vi "FTW_AppLauncher-Core_Config_Populate.vi"(0 "FTW-AppLauncher-Core In":refnum<class "FTW-AppLauncher-Core.lvclass">, 11 "error in":errorcluster) -> (4 "FTW-AppLauncher-Core Out":refnum<class "FTW-AppLauncher-Core.lvclass">, 6 "Configuration String":string, 15 "error out":errorcluster)   [LabVIEW 2013, in "FTW-AppLauncher-Core.lvclass"]
uses:
  FTW-AppLauncher-Core.lvclass
  source/JSON/FTW-JSON-UpdateMode.ctl
  FTW-AppLauncher-Core.lvclass/FTW-AppLauncher-Core.ctl
  source/JSON/FTW-JSON.lvclass
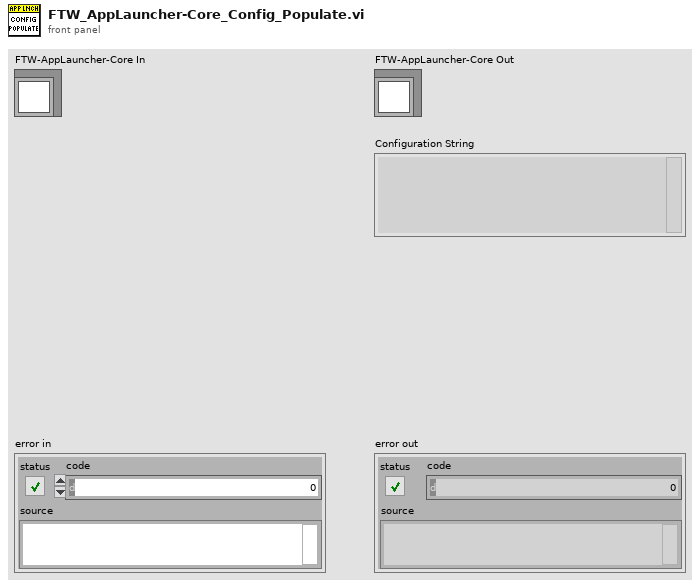
[diagram p1: front panel]
types:
  T1 = typedef "FTW-JSON.lvclass/FTW-JSON-UpdateMode.ctl" = enum16{"Upsert", "Update Only", "Insert Only"}
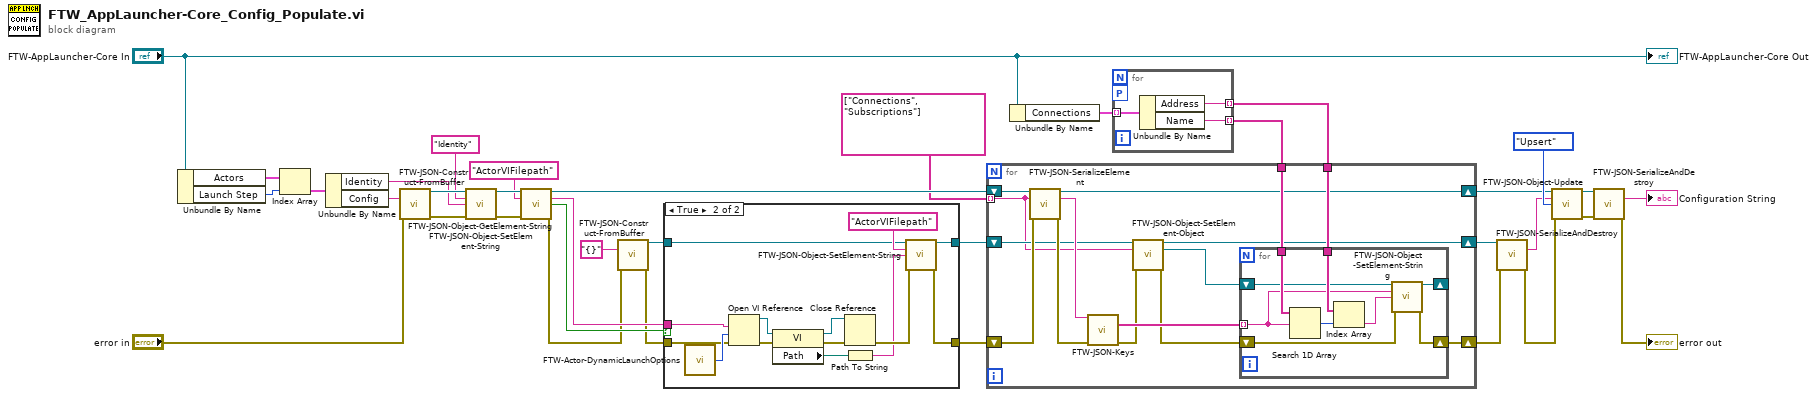
[diagram p0: block diagram]
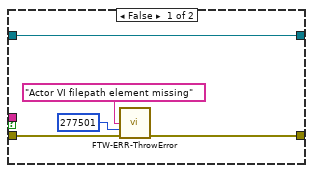
[diagram p2: hidden frame]
diagram:
  n1 = Unbundle By Name("FTW-AppLauncher-Core In") -> ("Actors"=w36:cluster{"Identity":string, "Config":string}[], "Launch Step"=w35:i32)
  n2 = Index Array(array=w36, index=w35) -> (element=w34:cluster{"Identity":string, "Config":string})
  n3 = Unbundle By Name(w34) -> ("Identity"=w30:string, "Config"=w22:string)
  n4 = call "FTW-JSON-Construct-FromBuffer.vi"("JSON String (UTF-8)"=w22, "error in"="error in") -> ("JSON Object"=w33:refnum<class "FTW-JSON.lvclass">, "error out"=w32:errorcluster)  [unwired: 12 in]
  n5 = call "FTW-JSON-Object-SetElement-String.vi"("JSON Object"=w33, "Key"="Identity", "Value"=w30, "error in"=w32) -> ("JSON Object out"=w29:refnum<class "FTW-JSON.lvclass">, "error out"=w28:errorcluster)  [unwired: 10 in]
  n6 = call "FTW-JSON-Object-GetElement-String.vi"("JSON Object"=w29, "Key"="ActorVIFilepath", "error in"=w28) -> ("JSON Object out"=w20:refnum<class "FTW-JSON.lvclass">, "Value"=w26:string, "Found?"=w21:bool, "error out"=w6:errorcluster)  [unwired: 9 in]
  n7 = call "FTW-JSON-Construct-FromBuffer.vi"("JSON String (UTF-8)"="{}", "error in"=w6) -> ("JSON Object"=w7:refnum<class "FTW-JSON.lvclass">, "error out"=w5:errorcluster)  [unwired: 12 in]
  n8 = case shown="True" w21 {
    tunnel: w26 -> [_ w49]
    tunnel: [w37 w43] -> w17
    tunnel: [w38 w44] -> w23
    tunnel: w5 -> [w39 w45]
    tunnel: w7 -> [w37 w42]
    frame False {
      n9 = call "FTW-ERR-ThrowError.vi"("Error Message"="Actor VI filepath element missing", "Error Code"=277501, "error in"=w39) -> ("error out"=w38:errorcluster)  [unwired: 12 in]
    }
    frame True {
      n10 = call "FTW-Actor-DynamicLaunchOptions.vi"() -> ("Open VI Ref Options"=w55:i32)
      n11 = Open VI Reference(vi path=w49, options=w55, error in (no error)=w45) -> (vi reference=w52:refnum<vi>, error out=w54:errorcluster)  [unwired: 3 in]
      n12 = property class="VI"(reference=w52, error in=w54) -> (reference out=w51:refnum<vi>, error out=w53:errorcluster, "Path"=w50:path)
      n13 = Close Reference(reference=w51, error in (no error)=w53) -> (error out=w48:errorcluster)
      n14 = Path To String(path=w50) -> (string=w46:string)
      n15 = call "FTW-JSON-Object-SetElement-String.vi"("JSON Object"=w42, "Key"="ActorVIFilepath", "Value"=w46, "error in"=w48) -> ("JSON Object out"=w43:refnum<class "FTW-JSON.lvclass">, "error out"=w44:errorcluster)  [unwired: 10 in]
    }
  }
  n16 = Unbundle By Name("FTW-AppLauncher-Core In") -> ("Connections"=w18:cluster{"Name":string, "Address":string}[])
  n17 = for {
    tunnel: w18 -> [w58] mode=indexing
    workers-P: _ -> [_]
    tunnel: [w57] -> w15 mode=indexing
    tunnel: [w56] -> w16 mode=indexing
    n18 = Unbundle By Name(w58) -> ("Address"=w56:string, "Name"=w57:string)
  }
  n19 = for {
    tunnel: string[] ["Connections", "Subscriptions"] -> [w61] mode=indexing
    tunnel: w16 -> [w67]
    tunnel: w15 -> [w66]
    shift-right: [w59] -> w4
    shift-left: w17 -> [w62]
    shift-right: [w64] -> w3
    shift-left: w23 -> [w73]
    shift-right: [w65] -> w14
    shift-left: w20 -> [w71]
    n20 = call "FTW-JSON-SerializeElement.vi"("JSON Object"=w71, "Key"=w61, "error in"=w73) -> ("JSON Object"=w65:refnum<class "FTW-JSON.lvclass">, "Element as JSON String"=w70:string, "error out"=w72:errorcluster)  [unwired: 9 in, 1 out]
    n21 = call "FTW-JSON-Keys.vi"("JSON Opject"=w70, "error in"=w72) -> ("Keys"=w69:string[], "error out"=w68:errorcluster)  [unwired: 11 in, 1 out]
    n22 = call "FTW-JSON-Object-SetElement-Object.vi"("JSON Object"=w62, "Key"=w61, "error in"=w68) -> ("JSON Root Object"=w59:refnum<class "FTW-JSON.lvclass">, "JSON Sub-Object"=w60:refnum<class "FTW-JSON.lvclass">, "error out"=w63:errorcluster)  [unwired: 10 in]
    n23 = for {
      tunnel: w66 -> [w82]
      tunnel: w69 -> [w79] mode=indexing
      tunnel: w67 -> [w80]
      shift-right: [w77] -> _
      shift-left: w60 -> [w74]
      shift-right: [w75] -> w64
      shift-left: w63 -> [w76]
      n24 = Search 1D Array(1D array=w82, element=w79) -> (index of element=w81:i32)  [unwired: 1 in]
      n25 = Index Array(array=w80, index=w81) -> (element=w78:string)
      n26 = call "FTW-JSON-Object-SetElement-String.vi"("JSON Object"=w74, "Key"=w79, "Value"=w78, "error in"=w76) -> ("JSON Object out"=w77:refnum<class "FTW-JSON.lvclass">, "error out"=w75:errorcluster)  [unwired: 10 in]
    }
  }
  n27 = call "FTW-JSON-SerializeAndDestroy.vi"("JSON Object"=w4, "error in"=w3) -> ("JSON String (UTF-8)"=w1:string, "error out"=w2:errorcluster)  [unwired: 12 in]
  n28 = call "FTW-JSON-Object-Update.vi"("JSON Object"=w14, "JSON Object to Merge"=w1, "Update Mode"=FTW-JSON-UpdateMode."Upsert", "error in"=w2) -> ("JSON Object out"=w12:refnum<class "FTW-JSON.lvclass">, "error out"=w13:errorcluster)  [unwired: 10 in]
  n29 = call "FTW-JSON-SerializeAndDestroy.vi"("JSON Object"=w12, "error in"=w13) -> ("JSON String (UTF-8)"=→"Configuration String":string, "error out"=→"error out":errorcluster)  [unwired: 12 in]
  "FTW-AppLauncher-Core Out" <- "FTW-AppLauncher-Core In"
